vi "TesterOption (SubVI).vi"(5 "On/Off 2":bool=TRUE, 6 "Tester Option 2":T1(ring), 7 "2 Options":bool, 8 "error in (no error)":errorcluster, 9 "On/Off":bool=TRUE, 10 "Tester Option":T1(ring), 11 "VISA Refnum in":refnum<visa-resource-name>) -> (0 "error out":errorcluster, 3 "VISA Refnum out":refnum<visa-resource-name>)   [LabVIEW 2017]
panel:
  out "x .or. y?":u8[](array[numeric])
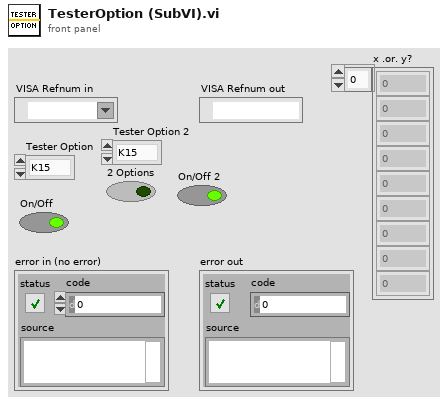
[diagram p1: front panel]
types:
  T1 = enum16{"K15", "K16", "K17", "Venable", "Firmeware", "Fan", "Power", "120C", "110C", "100C", "90C", "80C", "70C", "60C", "50C", "40C", "30C", "25C", "20C", "10C", "0C"}
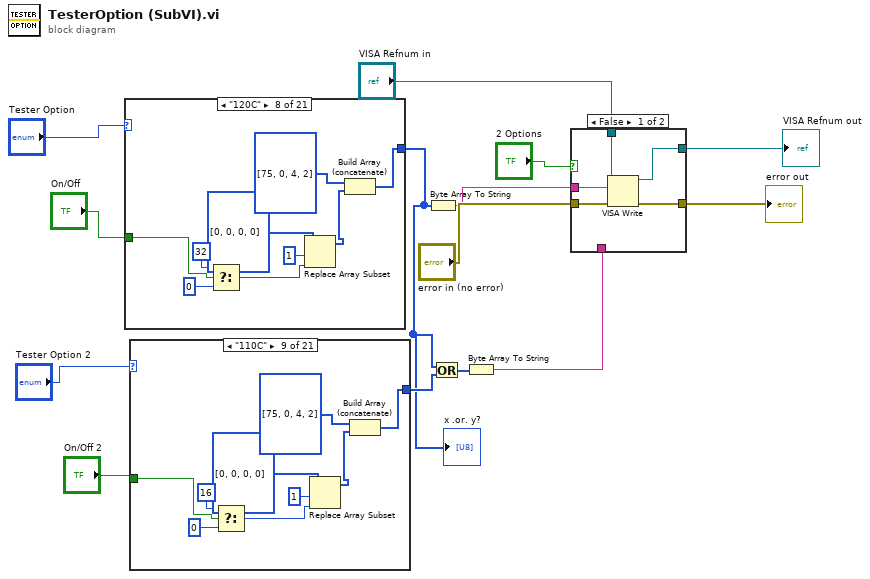
[diagram p0: block diagram]
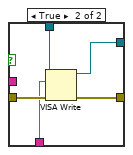
[diagram p2: hidden frame]
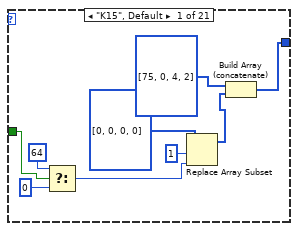
[diagram p3: hidden frame]
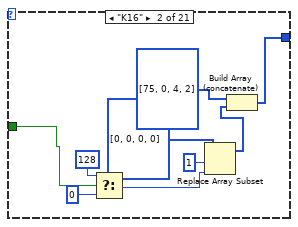
[diagram p4: hidden frame]
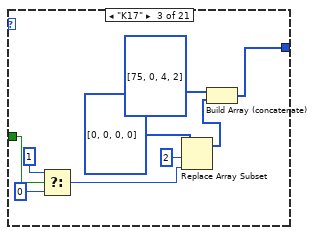
[diagram p5: hidden frame]
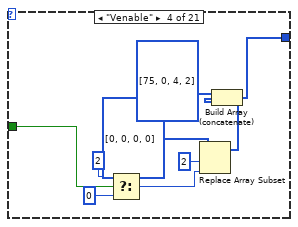
[diagram p6: hidden frame]
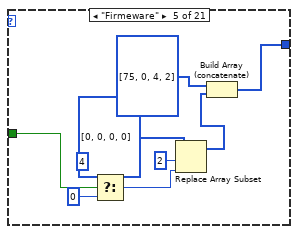
[diagram p7: hidden frame]
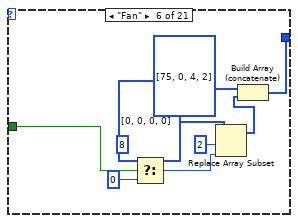
[diagram p8: hidden frame]
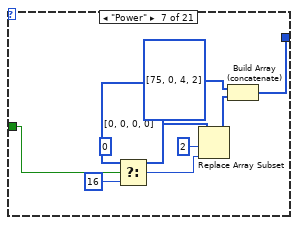
[diagram p9: hidden frame]
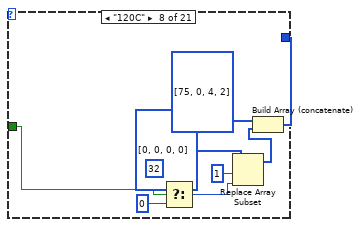
[diagram p10: hidden frame]
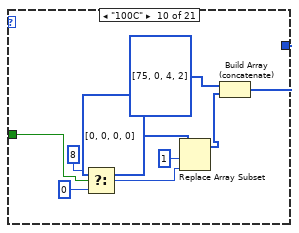
[diagram p11: hidden frame]
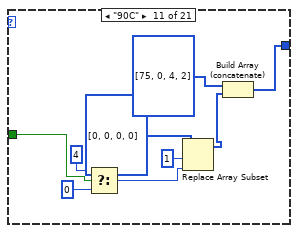
[diagram p12: hidden frame]
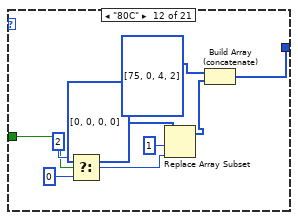
[diagram p13: hidden frame]
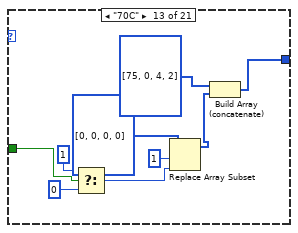
[diagram p14: hidden frame]
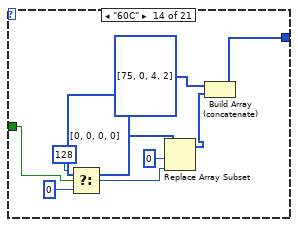
[diagram p15: hidden frame]
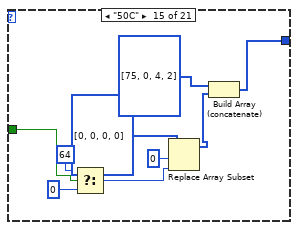
[diagram p16: hidden frame]
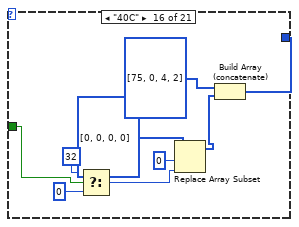
[diagram p17: hidden frame]
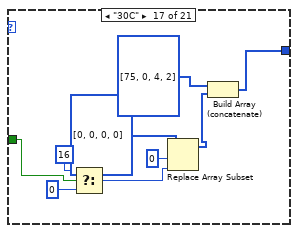
[diagram p18: hidden frame]
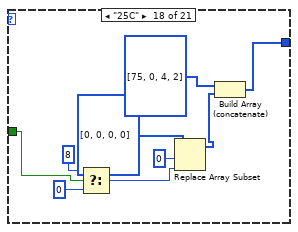
[diagram p19: hidden frame]
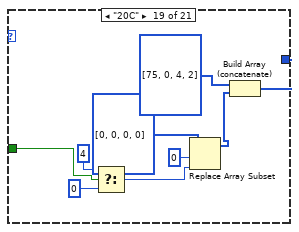
[diagram p20: hidden frame]
diagram:
  n1 = case shown="\"120C\"" "Tester Option" {
    tunnel: [w22 w31 w33 w49 w58 w67 w75 w79 w87 w97 w106 w115 w123 w133 w142 w151 w160 w169 w178 w187 w196] -> w1
    tunnel: "On/Off" -> [w16 w25 w34 w43 w52 w61 w71 w78 w88 w96 w105 w114 w124 w132 w141 w150 w159 w168 w177 w186 w195]
    frame "K15", Default {
      n2 = Select(t=u8 64, s=w16, f=u8 0) -> (s? t:f=w17:u8)
      n3 = Replace Array Subset(array=u8[] [0, 0, 0, 0], new element=w17, index=1) -> (w15:u8[])
      n4 = Build Array (concatenate)(u8[] [75, 0, 4, 2], w15) -> (w22:u8[])
    }
    frame "K16" {
      n5 = Select(t=u8 128, s=w25, f=u8 0) -> (s? t:f=w26:u8)
      n6 = Replace Array Subset(array=u8[] [0, 0, 0, 0], new element=w26, index=1) -> (w24:u8[])
      n7 = Build Array (concatenate)(u8[] [75, 0, 4, 2], w24) -> (w31:u8[])
    }
    frame "K17" {
      n8 = Select(t=u8 1, s=w34, f=u8 0) -> (s? t:f=w36:u8)
      n9 = Replace Array Subset(array=u8[] [0, 0, 0, 0], new element=w36, index=2) -> (w35:u8[])
      n10 = Build Array (concatenate)(u8[] [75, 0, 4, 2], w35) -> (w33:u8[])
    }
    frame "Venable" {
      n11 = Select(t=u8 2, s=w43, f=u8 0) -> (s? t:f=w44:u8)
      n12 = Replace Array Subset(array=u8[] [0, 0, 0, 0], new element=w44, index=2) -> (w42:u8[])
      n13 = Build Array (concatenate)(u8[] [75, 0, 4, 2], w42) -> (w49:u8[])
    }
    frame "Firmeware" {
      n14 = Select(t=u8 4, s=w52, f=u8 0) -> (s? t:f=w53:u8)
      n15 = Replace Array Subset(array=u8[] [0, 0, 0, 0], new element=w53, index=2) -> (w51:u8[])
      n16 = Build Array (concatenate)(u8[] [75, 0, 4, 2], w51) -> (w58:u8[])
    }
    frame "Fan" {
      n17 = Select(t=u8 8, s=w61, f=u8 0) -> (s? t:f=w62:u8)
      n18 = Replace Array Subset(array=u8[] [0, 0, 0, 0], new element=w62, index=2) -> (w60:u8[])
      n19 = Build Array (concatenate)(u8[] [75, 0, 4, 2], w60) -> (w67:u8[])
    }
    frame "Power" {
      n20 = Select(t=u8 0, s=w71, f=u8 16) -> (s? t:f=w69:u8)
      n21 = Replace Array Subset(array=u8[] [0, 0, 0, 0], new element=w69, index=2) -> (w74:u8[])
      n22 = Build Array (concatenate)(u8[] [75, 0, 4, 2], w74) -> (w75:u8[])
    }
    frame "120C" {
      n23 = Select(t=u8 32, s=w78, f=u8 0) -> (s? t:f=w81:u8)
      n24 = Replace Array Subset(array=u8[] [0, 0, 0, 0], new element=w81, index=1) -> (w80:u8[])
      n25 = Build Array (concatenate)(u8[] [75, 0, 4, 2], w80) -> (w79:u8[])
    }
    frame "110C" {
      n26 = Select(t=u8 16, s=w88, f=u8 0) -> (s? t:f=w90:u8)
      n27 = Replace Array Subset(array=u8[] [0, 0, 0, 0], new element=w90, index=1) -> (w89:u8[])
      n28 = Build Array (concatenate)(u8[] [75, 0, 4, 2], w89) -> (w87:u8[])
    }
    frame "100C" {
      n29 = Select(t=u8 8, s=w96, f=u8 0) -> (s? t:f=w99:u8)
      n30 = Replace Array Subset(array=u8[] [0, 0, 0, 0], new element=w99, index=1) -> (w98:u8[])
      n31 = Build Array (concatenate)(u8[] [75, 0, 4, 2], w98) -> (w97:u8[])
    }
    frame "90C" {
      n32 = Select(t=u8 4, s=w105, f=u8 0) -> (s? t:f=w108:u8)
      n33 = Replace Array Subset(array=u8[] [0, 0, 0, 0], new element=w108, index=1) -> (w107:u8[])
      n34 = Build Array (concatenate)(u8[] [75, 0, 4, 2], w107) -> (w106:u8[])
    }
    frame "80C" {
      n35 = Select(t=u8 2, s=w114, f=u8 0) -> (s? t:f=w117:u8)
      n36 = Replace Array Subset(array=u8[] [0, 0, 0, 0], new element=w117, index=1) -> (w116:u8[])
      n37 = Build Array (concatenate)(u8[] [75, 0, 4, 2], w116) -> (w115:u8[])
    }
    frame "70C" {
      n38 = Select(t=u8 1, s=w124, f=u8 0) -> (s? t:f=w126:u8)
      n39 = Replace Array Subset(array=u8[] [0, 0, 0, 0], new element=w126, index=1) -> (w125:u8[])
      n40 = Build Array (concatenate)(u8[] [75, 0, 4, 2], w125) -> (w123:u8[])
    }
    frame "60C" {
      n41 = Select(t=u8 128, s=w132, f=u8 0) -> (s? t:f=w135:u8)
      n42 = Replace Array Subset(array=u8[] [0, 0, 0, 0], new element=w135, index=0) -> (w134:u8[])
      n43 = Build Array (concatenate)(u8[] [75, 0, 4, 2], w134) -> (w133:u8[])
    }
    frame "50C" {
      n44 = Select(t=u8 64, s=w141, f=u8 0) -> (s? t:f=w144:u8)
      n45 = Replace Array Subset(array=u8[] [0, 0, 0, 0], new element=w144, index=0) -> (w143:u8[])
      n46 = Build Array (concatenate)(u8[] [75, 0, 4, 2], w143) -> (w142:u8[])
    }
    frame "40C" {
      n47 = Select(t=u8 32, s=w150, f=u8 0) -> (s? t:f=w153:u8)
      n48 = Replace Array Subset(array=u8[] [0, 0, 0, 0], new element=w153, index=0) -> (w152:u8[])
      n49 = Build Array (concatenate)(u8[] [75, 0, 4, 2], w152) -> (w151:u8[])
    }
    frame "30C" {
      n50 = Select(t=u8 16, s=w159, f=u8 0) -> (s? t:f=w162:u8)
      n51 = Replace Array Subset(array=u8[] [0, 0, 0, 0], new element=w162, index=0) -> (w161:u8[])
      n52 = Build Array (concatenate)(u8[] [75, 0, 4, 2], w161) -> (w160:u8[])
    }
    frame "25C" {
      n53 = Select(t=u8 8, s=w168, f=u8 0) -> (s? t:f=w171:u8)
      n54 = Replace Array Subset(array=u8[] [0, 0, 0, 0], new element=w171, index=0) -> (w170:u8[])
      n55 = Build Array (concatenate)(u8[] [75, 0, 4, 2], w170) -> (w169:u8[])
    }
    frame "20C" {
      n56 = Select(t=u8 4, s=w177, f=u8 0) -> (s? t:f=w180:u8)
      n57 = Replace Array Subset(array=u8[] [0, 0, 0, 0], new element=w180, index=0) -> (w179:u8[])
      n58 = Build Array (concatenate)(u8[] [75, 0, 4, 2], w179) -> (w178:u8[])
    }
    frame "10C" {
      n59 = Select(t=u8 2, s=w186, f=u8 0) -> (s? t:f=w189:u8)
      n60 = Replace Array Subset(array=u8[] [0, 0, 0, 0], new element=w189, index=0) -> (w188:u8[])
      n61 = Build Array (concatenate)(u8[] [75, 0, 4, 2], w188) -> (w187:u8[])
    }
    frame "0C" {
      n62 = Select(t=u8 1, s=w195, f=u8 0) -> (s? t:f=w198:u8)
      n63 = Replace Array Subset(array=u8[] [0, 0, 0, 0], new element=w198, index=0) -> (w197:u8[])
      n64 = Build Array (concatenate)(u8[] [75, 0, 4, 2], w197) -> (w196:u8[])
    }
  }
  "x .or. y?" <- w1
  n65 = case shown="\"110C\"" "Tester Option 2" {
    tunnel: [w211 w220 w222 w238 w247 w256 w264 w267 w277 w286 w295 w304 w312 w322 w331 w340 w349 w358 w367 w376 w385] -> w5
    tunnel: "On/Off 2" -> [w205 w214 w223 w232 w241 w250 w260 w268 w276 w285 w294 w303 w313 w321 w330 w339 w348 w357 w366 w375 w384]
    frame "K15", Default {
      n66 = Select(t=u8 64, s=w205, f=u8 0) -> (s? t:f=w206:u8)
      n67 = Replace Array Subset(array=u8[] [0, 0, 0, 0], new element=w206, index=1) -> (w204:u8[])
      n68 = Build Array (concatenate)(u8[] [75, 0, 4, 2], w204) -> (w211:u8[])
    }
    frame "K16" {
      n69 = Select(t=u8 128, s=w214, f=u8 0) -> (s? t:f=w215:u8)
      n70 = Replace Array Subset(array=u8[] [0, 0, 0, 0], new element=w215, index=1) -> (w213:u8[])
      n71 = Build Array (concatenate)(u8[] [75, 0, 4, 2], w213) -> (w220:u8[])
    }
    frame "K17" {
      n72 = Select(t=u8 1, s=w223, f=u8 0) -> (s? t:f=w225:u8)
      n73 = Replace Array Subset(array=u8[] [0, 0, 0, 0], new element=w225, index=2) -> (w224:u8[])
      n74 = Build Array (concatenate)(u8[] [75, 0, 4, 2], w224) -> (w222:u8[])
    }
    frame "Venable" {
      n75 = Select(t=u8 2, s=w232, f=u8 0) -> (s? t:f=w233:u8)
      n76 = Replace Array Subset(array=u8[] [0, 0, 0, 0], new element=w233, index=2) -> (w231:u8[])
      n77 = Build Array (concatenate)(u8[] [75, 0, 4, 2], w231) -> (w238:u8[])
    }
    frame "Firmeware" {
      n78 = Select(t=u8 4, s=w241, f=u8 0) -> (s? t:f=w242:u8)
      n79 = Replace Array Subset(array=u8[] [0, 0, 0, 0], new element=w242, index=2) -> (w240:u8[])
      n80 = Build Array (concatenate)(u8[] [75, 0, 4, 2], w240) -> (w247:u8[])
    }
    frame "Fan" {
      n81 = Select(t=u8 8, s=w250, f=u8 0) -> (s? t:f=w251:u8)
      n82 = Replace Array Subset(array=u8[] [0, 0, 0, 0], new element=w251, index=2) -> (w249:u8[])
      n83 = Build Array (concatenate)(u8[] [75, 0, 4, 2], w249) -> (w256:u8[])
    }
    frame "Power" {
      n84 = Select(t=u8 0, s=w260, f=u8 16) -> (s? t:f=w258:u8)
      n85 = Replace Array Subset(array=u8[] [0, 0, 0, 0], new element=w258, index=2) -> (w263:u8[])
      n86 = Build Array (concatenate)(u8[] [75, 0, 4, 2], w263) -> (w264:u8[])
    }
    frame "120C" {
      n87 = Select(t=u8 32, s=w268, f=u8 0) -> (s? t:f=w270:u8)
      n88 = Replace Array Subset(array=u8[] [0, 0, 0, 0], new element=w270, index=1) -> (w269:u8[])
      n89 = Build Array (concatenate)(u8[] [75, 0, 4, 2], w269) -> (w267:u8[])
    }
    frame "110C" {
      n90 = Select(t=u8 16, s=w276, f=u8 0) -> (s? t:f=w279:u8)
      n91 = Replace Array Subset(array=u8[] [0, 0, 0, 0], new element=w279, index=1) -> (w278:u8[])
      n92 = Build Array (concatenate)(u8[] [75, 0, 4, 2], w278) -> (w277:u8[])
    }
    frame "100C" {
      n93 = Select(t=u8 8, s=w285, f=u8 0) -> (s? t:f=w288:u8)
      n94 = Replace Array Subset(array=u8[] [0, 0, 0, 0], new element=w288, index=1) -> (w287:u8[])
      n95 = Build Array (concatenate)(u8[] [75, 0, 4, 2], w287) -> (w286:u8[])
    }
    frame "90C" {
      n96 = Select(t=u8 4, s=w294, f=u8 0) -> (s? t:f=w297:u8)
      n97 = Replace Array Subset(array=u8[] [0, 0, 0, 0], new element=w297, index=1) -> (w296:u8[])
      n98 = Build Array (concatenate)(u8[] [75, 0, 4, 2], w296) -> (w295:u8[])
    }
    frame "80C" {
      n99 = Select(t=u8 2, s=w303, f=u8 0) -> (s? t:f=w306:u8)
      n100 = Replace Array Subset(array=u8[] [0, 0, 0, 0], new element=w306, index=1) -> (w305:u8[])
      n101 = Build Array (concatenate)(u8[] [75, 0, 4, 2], w305) -> (w304:u8[])
    }
    frame "70C" {
      n102 = Select(t=u8 1, s=w313, f=u8 0) -> (s? t:f=w315:u8)
      n103 = Replace Array Subset(array=u8[] [0, 0, 0, 0], new element=w315, index=1) -> (w314:u8[])
      n104 = Build Array (concatenate)(u8[] [75, 0, 4, 2], w314) -> (w312:u8[])
    }
    frame "60C" {
      n105 = Select(t=u8 128, s=w321, f=u8 0) -> (s? t:f=w324:u8)
      n106 = Replace Array Subset(array=u8[] [0, 0, 0, 0], new element=w324, index=0) -> (w323:u8[])
      n107 = Build Array (concatenate)(u8[] [75, 0, 4, 2], w323) -> (w322:u8[])
    }
    frame "50C" {
      n108 = Select(t=u8 64, s=w330, f=u8 0) -> (s? t:f=w333:u8)
      n109 = Replace Array Subset(array=u8[] [0, 0, 0, 0], new element=w333, index=0) -> (w332:u8[])
      n110 = Build Array (concatenate)(u8[] [75, 0, 4, 2], w332) -> (w331:u8[])
    }
    frame "40C" {
      n111 = Select(t=u8 32, s=w339, f=u8 0) -> (s? t:f=w342:u8)
      n112 = Replace Array Subset(array=u8[] [0, 0, 0, 0], new element=w342, index=0) -> (w341:u8[])
      n113 = Build Array (concatenate)(u8[] [75, 0, 4, 2], w341) -> (w340:u8[])
    }
    frame "30C" {
      n114 = Select(t=u8 16, s=w348, f=u8 0) -> (s? t:f=w351:u8)
      n115 = Replace Array Subset(array=u8[] [0, 0, 0, 0], new element=w351, index=0) -> (w350:u8[])
      n116 = Build Array (concatenate)(u8[] [75, 0, 4, 2], w350) -> (w349:u8[])
    }
    frame "25C" {
      n117 = Select(t=u8 8, s=w357, f=u8 0) -> (s? t:f=w360:u8)
      n118 = Replace Array Subset(array=u8[] [0, 0, 0, 0], new element=w360, index=0) -> (w359:u8[])
      n119 = Build Array (concatenate)(u8[] [75, 0, 4, 2], w359) -> (w358:u8[])
    }
    frame "20C" {
      n120 = Select(t=u8 4, s=w366, f=u8 0) -> (s? t:f=w369:u8)
      n121 = Replace Array Subset(array=u8[] [0, 0, 0, 0], new element=w369, index=0) -> (w368:u8[])
      n122 = Build Array (concatenate)(u8[] [75, 0, 4, 2], w368) -> (w367:u8[])
    }
    frame "10C" {
      n123 = Select(t=u8 2, s=w375, f=u8 0) -> (s? t:f=w378:u8)
      n124 = Replace Array Subset(array=u8[] [0, 0, 0, 0], new element=w378, index=0) -> (w377:u8[])
      n125 = Build Array (concatenate)(u8[] [75, 0, 4, 2], w377) -> (w376:u8[])
    }
    frame "0C" {
      n126 = Select(t=u8 1, s=w384, f=u8 0) -> (s? t:f=w387:u8)
      n127 = Replace Array Subset(array=u8[] [0, 0, 0, 0], new element=w387, index=0) -> (w386:u8[])
      n128 = Build Array (concatenate)(u8[] [75, 0, 4, 2], w386) -> (w385:u8[])
    }
  }
  n129 = Byte Array To String(unsigned byte array=w1) -> (string=w10:string)
  n130 = Or(x=w1, y=w5) -> (x .or. y?=w4:u8[])
  n131 = Byte Array To String(unsigned byte array=w4) -> (string=w2:string)
  n132 = case shown="False" "2 Options" {
    tunnel: [w397 w402] -> w14
    tunnel: "error in (no error)" -> [w396 w401]
    tunnel: [w395 w400] -> w12
    tunnel: "VISA Refnum in" -> [w394 w399]
    tunnel: w10 -> [w393 _]
    tunnel: w2 -> [_ w398]
    frame False {
      n133 = VISA Write(VISA resource name=w394, write buffer=w393, error in (no error)=w396) -> (VISA resource name out=w395:refnum<visa-resource-name>, error out=w397:errorcluster)  [unwired: 1 out]
    }
    frame True {
      n134 = VISA Write(VISA resource name=w399, write buffer=w398, error in (no error)=w401) -> (VISA resource name out=w400:refnum<visa-resource-name>, error out=w402:errorcluster)  [unwired: 1 out]
    }
  }
  "VISA Refnum out" <- w12
  "error out" <- w14
